vi "mapClassNameToGObjectEnum.vi"(8 "error in (no error)":errorcluster, 10 "Class Name":string, 11 "Project in":refnum<class "Project.lvclass">) -> (0 "error out":errorcluster, 2 "GObjectSelection":T1, 3 "Project out":refnum<class "Project.lvclass">)   [LabVIEW 2016, in "Project.lvclass"]
uses:
  Project.lvclass
  Typedefs/GObjectSelection.ctl
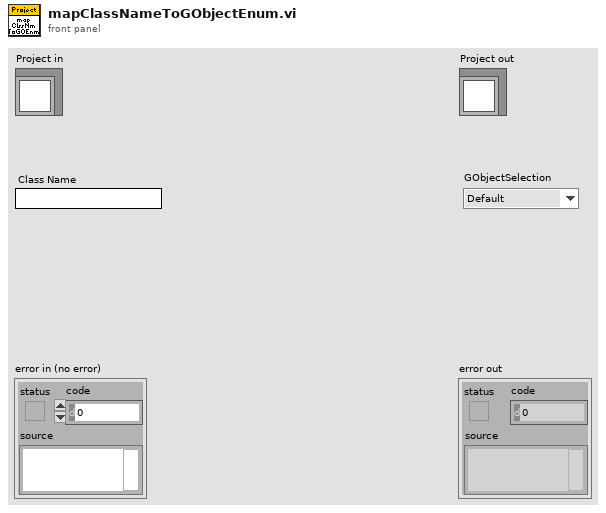
[diagram p1: front panel]
types:
  T1 = typedef "GObjectSelection.ctl" = enum16{"Default", "ClusterConstant", "EnumConstant"}
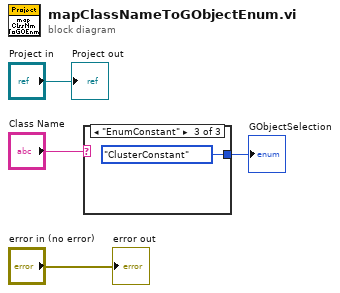
[diagram p0: block diagram]
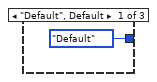
[diagram p2: hidden frame]
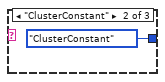
[diagram p3: hidden frame]
diagram:
  n1 = case shown="\"EnumConstant\"" "Class Name" {
    tunnel: [GObjectSelection."Default" ("DiagramObjectSelection") GObjectSelection."ClusterConstant" ("DiagramObjectSelection") GObjectSelection."ClusterConstant" ("DiagramObjectSelection")] -> w1
    frame "Default", Default {
    }
    frame "ClusterConstant" {
    }
    frame "EnumConstant" {
    }
  }
  "GObjectSelection" <- w1
  "error out" <- "error in (no error)"
  "Project out" <- "Project in"
